vi "JSON Numeric Probe.vi"(11 "JSON out":refnum<class "JSON Numeric.lvclass">) -> (2 "Value String":string, 3 "Boolean":bool)   [LabVIEW 2017]
uses:
  JSON Numeric.lvclass
  Read value (Numeric).vi
panel:
  out "value":dbl
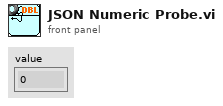
[diagram p1: front panel]
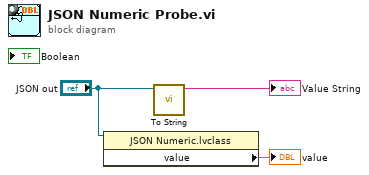
[diagram p0: block diagram]
diagram:
  n1 = property class="JSON Numeric.lvclass"(reference="JSON out") -> ("value"=→"value":dbl)  [unwired: 1 in, 2 out]
  n2 = call-dynamic "To String.vi"("JSON Numeric in"="JSON out") -> ("String"=→"Value String":string)  [unwired: 9 in, 1 out]
